vi "normBit.vi"(9 "method":T1(ring), 11 "Rxy":dbl[][](array[numeric])) -> (1 "standard deviation":dbl format="%0.2f", 3 "Array":dbl[][](array[numeric]))   [LabVIEW 2021]
uses:
  <vilib>/Analysis/baseanly.llb/Mean (DBL).vi
  <vilib>/Analysis/NI_AALBase.lvlib
  <vilib>/Analysis/NI_AALPro.lvlib
panel:
  out "Array 3":dbl[](array[numeric])
  out "Array 2":dbl[](array[numeric])
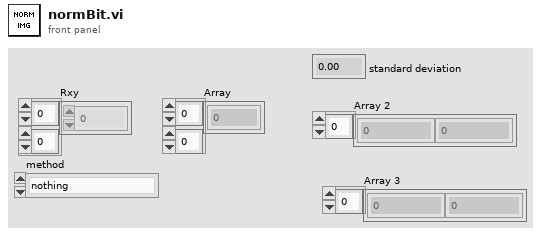
[diagram p1: front panel]
types:
  T1 = enum16{"nothing", "average", "8bit", "average/plane", "minimum", "plane", "average/stddev", "plane/average", "slope"}
  T2 = enum16{"nothing", "average", "8bit", "average/plane", "minimum", "plane", "average/stddev", "plane/average"}
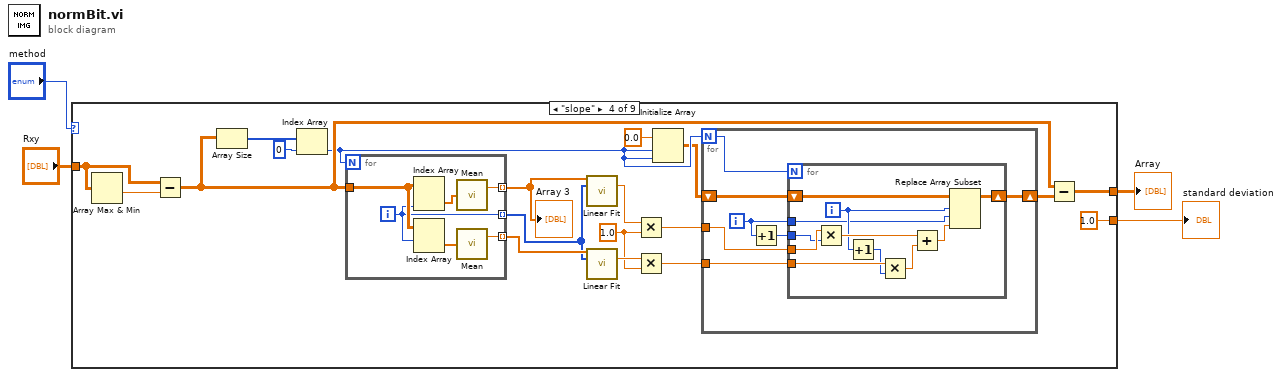
[diagram p0: block diagram]
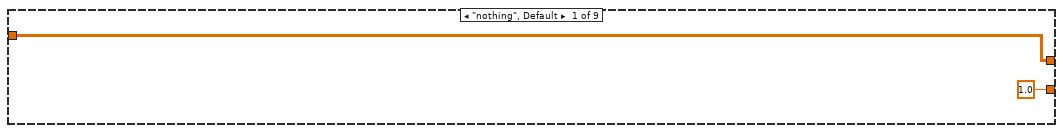
[diagram p2: hidden frame]
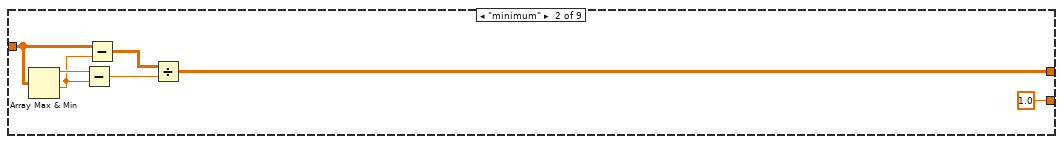
[diagram p3: hidden frame]
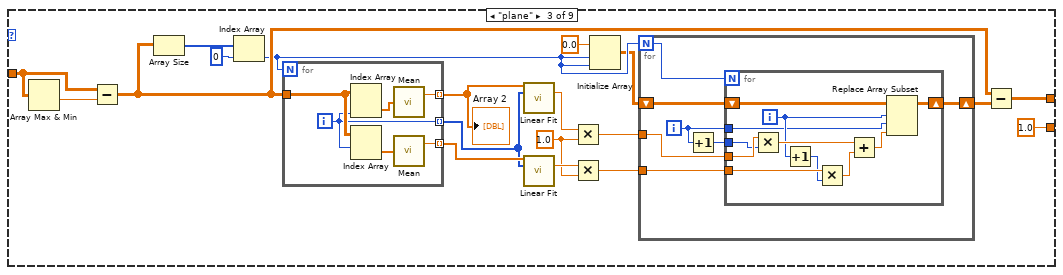
[diagram p4: hidden frame]
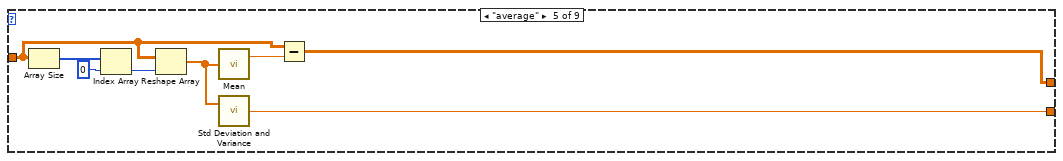
[diagram p5: hidden frame]
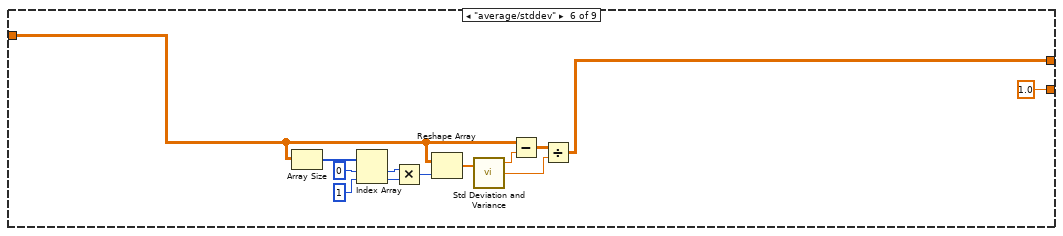
[diagram p6: hidden frame]
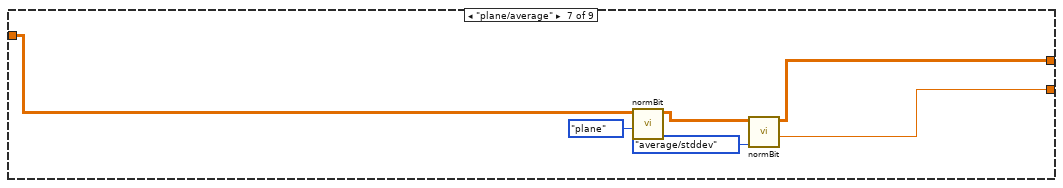
[diagram p7: hidden frame]
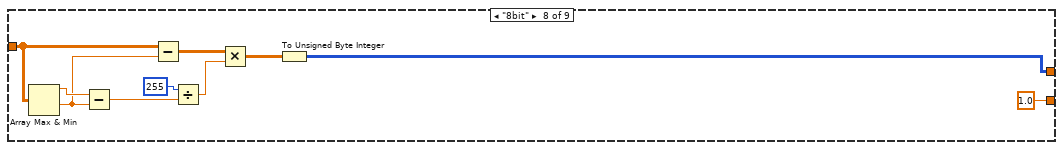
[diagram p8: hidden frame]
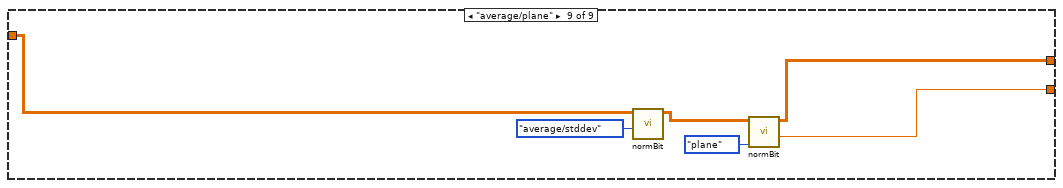
[diagram p9: hidden frame]
diagram:
  n1 = case shown="\"slope\"" "method" {
    tunnel: [w6 w8 w32 w75 w104 w109 w124 w128 w140] -> w4
    tunnel: "Rxy" -> [w6 w13 w24 w67 w103 w108 w126 w129 w142]
    tunnel: [1.0 ("standard deviation") 1.0 ("standard deviation") 1.0 ("standard deviation") 1.0 ("standard deviation") w100 1.0 ("standard deviation") w123 1.0 ("standard deviation") w139] -> w2
    frame "nothing", Default {
    }
    frame "minimum" {
      n2 = Array Max & Min(array=w13) -> (max value=w12:dbl, min value=w11:dbl)  [unwired: 2 out]
      n3 = Subtract(x=w12, y=w11) -> (x-y=w9:dbl)
      n4 = Subtract(x=w13, y=w11) -> (x-y=w10:dbl[][])
      n5 = Divide(x=w10, y=w9) -> (x/y=w8:dbl[][])
    }
    frame "plane" {
      w19 = 1.0 ("y")
      n6 = Array Max & Min(array=w24) -> (min value=w22:dbl)  [unwired: 3 out]
      n7 = Subtract(x=w24, y=w22) -> (x-y=w23:dbl[][])
      n8 = Array Size(array=w23) -> (size(s)=w31:i32[])
      n9 = Index Array(array=w31, index=0) -> (element=w17:i32)
      n10 = for {
        N: w17 -> [_]
        tunnel: w23 -> [w56]
        tunnel: [w51] -> w27 mode=indexing
        tunnel: [w53] -> w29 mode=indexing
        tunnel: [w52] -> w28 mode=indexing
        i -> [w51]
        n11 = Index Array(array=w56, index (col)=w51) -> (element=w54:dbl[])  [unwired: 1 in]
        n12 = Index Array(array=w56, index (row)=w51) -> (element=w55:dbl[])  [unwired: 1 in]
        n13 = call-poly <vilib>:"Mean.vi"("X"=w54) -> ("mean"=w52:dbl)  [unwired: 1 out]
        n14 = call-poly <vilib>:"Mean.vi"("X"=w55) -> ("mean"=w53:dbl)  [unwired: 1 out]
      }
      "Array 2" <- w28
      n15 = call <vilib>:"Linear Fit.vi"("Y"=w28, "X"=w27) -> ("slope"=w25:dbl)  [unwired: 9 in, 4 out]
      n16 = call <vilib>:"Linear Fit.vi"("Y"=w29, "X"=w27) -> ("slope"=w26:dbl)  [unwired: 9 in, 4 out]
      n17 = Multiply(x=w25, y=w19) -> (x*y=w21:dbl)
      n18 = Multiply(x=w26, y=w19) -> (x*y=w20:dbl)
      n19 = Initialize Array(0.0 ("element"), w17, w17) -> (w15:dbl[][])
      n20 = for {
        N: w17 -> [w35]
        tunnel: w20 -> [w39]
        tunnel: w21 -> [w38]
        shift-right: [w37] -> w14
        shift-left: w15 -> [w36]
        i -> [w33]
        n21 = Increment(x=w33) -> (x+1=w34:i32)
        n22 = for {
          N: w35 -> [_]
          tunnel: w39 -> [w50]
          tunnel: w38 -> [w49]
          shift-right: [w45] -> w37
          shift-left: w36 -> [w44]
          tunnel: w34 -> [w43]
          tunnel: w33 -> [w40]
          i -> [w41]
          n23 = Multiply(x=w49, y=w43) -> (x*y=w46:dbl)
          n24 = Increment(x=w41) -> (x+1=w48:i32)
          n25 = Multiply(x=w50, y=w48) -> (x*y=w47:dbl)
          n26 = Add(x=w46, y=w47) -> (x+y=w42:dbl)
          n27 = Replace Array Subset(array=w44, new element=w42, index (row)=w41, index (col)=w40) -> (w45:dbl[][])
        }
      }
      n28 = Subtract(x=w23, y=w14) -> (x-y=w32:dbl[][])
    }
    frame "slope" {
      w62 = 1.0 ("y")
      n29 = Array Max & Min(array=w67) -> (min value=w65:dbl)  [unwired: 3 out]
      n30 = Subtract(x=w67, y=w65) -> (x-y=w66:dbl[][])
      n31 = Array Size(array=w66) -> (size(s)=w74:i32[])
      n32 = Index Array(array=w74, index=0) -> (element=w60:i32)
      n33 = for {
        N: w60 -> [_]
        tunnel: w66 -> [w99]
        tunnel: [w94] -> w70 mode=indexing
        tunnel: [w96] -> w72 mode=indexing
        tunnel: [w95] -> w71 mode=indexing
        i -> [w94]
        n34 = Index Array(array=w99, index (col)=w94) -> (element=w97:dbl[])  [unwired: 1 in]
        n35 = Index Array(array=w99, index (row)=w94) -> (element=w98:dbl[])  [unwired: 1 in]
        n36 = call-poly <vilib>:"Mean.vi"("X"=w97) -> ("mean"=w95:dbl)  [unwired: 1 out]
        n37 = call-poly <vilib>:"Mean.vi"("X"=w98) -> ("mean"=w96:dbl)  [unwired: 1 out]
      }
      "Array 3" <- w71
      n38 = call <vilib>:"Linear Fit.vi"("Y"=w71, "X"=w70) -> ("slope"=w68:dbl)  [unwired: 9 in, 4 out]
      n39 = call <vilib>:"Linear Fit.vi"("Y"=w72, "X"=w70) -> ("slope"=w69:dbl)  [unwired: 9 in, 4 out]
      n40 = Multiply(x=w68, y=w62) -> (x*y=w64:dbl)
      n41 = Multiply(x=w69, y=w62) -> (x*y=w63:dbl)
      n42 = Initialize Array(0.0 ("element"), w60, w60) -> (w58:dbl[][])
      n43 = for {
        N: w60 -> [w78]
        tunnel: w63 -> [w82]
        tunnel: w64 -> [w81]
        shift-right: [w80] -> w57
        shift-left: w58 -> [w79]
        i -> [w76]
        n44 = Increment(x=w76) -> (x+1=w77:i32)
        n45 = for {
          N: w78 -> [_]
          tunnel: w82 -> [w93]
          tunnel: w81 -> [w92]
          shift-right: [w88] -> w80
          shift-left: w79 -> [w87]
          tunnel: w77 -> [w86]
          tunnel: w76 -> [w83]
          i -> [w84]
          n46 = Multiply(x=w92, y=w86) -> (x*y=w89:dbl)
          n47 = Increment(x=w84) -> (x+1=w91:i32)
          n48 = Multiply(x=w93, y=w91) -> (x*y=w90:dbl)
          n49 = Add(x=w89, y=w90) -> (x+y=w85:dbl)
          n50 = Replace Array Subset(array=w87, new element=w85, index (row)=w84, index (col)=w83) -> (w88:dbl[][])
        }
      }
      n51 = Subtract(x=w66, y=w57) -> (x-y=w75:dbl[][])
    }
    frame "average" {
      n52 = Array Size(array=w103) -> (size(s)=w107:i32[])
      n53 = Index Array(array=w107, index=0) -> (element=w105:i32)
      n54 = Reshape Array(w103, w105) -> (w101:dbl[])
      n55 = call-poly <vilib>:"Mean.vi"("X"=w101) -> ("mean"=w102:dbl)  [unwired: 1 out]
      n56 = call <vilib>:"Std Deviation and Variance.vi"("X"=w101) -> ("standard deviation"=w100:dbl)  [unwired: 1 in, 2 out]
      n57 = Subtract(x=w103, y=w102) -> (x-y=w104:dbl[][])
    }
    frame "average/stddev" {
      n58 = Array Size(array=w108) -> (size(s)=w115:i32[])
      n59 = Index Array(array=w115, index #1=0 ("index"), index #2=1 ("index")) -> (element #1=w114:i32, element #2=w118:i32)
      n60 = Multiply(x=w114, y=w118) -> (x*y=w119:i32)
      n61 = Reshape Array(w108, w119) -> (w110:dbl[])
      n62 = call <vilib>:"Std Deviation and Variance.vi"("X"=w110) -> ("mean"=w111:dbl, "standard deviation"=w113:dbl)  [unwired: 1 in, 1 out]
      n63 = Subtract(x=w108, y=w111) -> (x-y=w112:dbl[][])
      n64 = Divide(x=w112, y=w113) -> (x/y=w109:dbl[][])
    }
    frame "plane/average" {
      n65 = call "normBit.vi"("method"=T2."plane", "Rxy"=w126) -> ("Array"=w125:dbl[][])  [unwired: 8 in, 1 out]
      n66 = call "normBit.vi"("method"=T2."average/stddev", "Rxy"=w125) -> ("standard deviation"=w123:dbl, "Array"=w124:dbl[][])  [unwired: 8 in]
    }
    frame "8bit" {
      n67 = Array Max & Min(array=w129) -> (max value=w132:dbl, min value=w131:dbl)  [unwired: 2 out]
      n68 = Subtract(x=w132, y=w131) -> (x-y=w134:dbl)
      n69 = Subtract(x=w129, y=w131) -> (x-y=w133:dbl[][])
      n70 = Divide(x=u8 255, y=w134) -> (x/y=w135:dbl)
      n71 = Multiply(x=w133, y=w135) -> (x*y=w130:dbl[][])
      n72 = To Unsigned Byte Integer(number=w130) -> (unsigned 8bit integer=w128:u8[][])
    }
    frame "average/plane" {
      n73 = call "normBit.vi"("method"=T2."average/stddev", "Rxy"=w142) -> ("Array"=w141:dbl[][])  [unwired: 8 in, 1 out]
      n74 = call "normBit.vi"("method"=T2."plane", "Rxy"=w141) -> ("standard deviation"=w139:dbl, "Array"=w140:dbl[][])  [unwired: 8 in]
    }
  }
  "Array" <- w4
  "standard deviation" <- w2
